vi "PH_Sequencer_Watch.PC _SetVoltage.vi"(0 "i ref in":refnum<vi>, 2 "Tagname":string, 3 "Tagvalue":dbl, 5 "error in (no error)":errorcluster) -> (14 "i ref out":refnum<vi>, 19 "error out":errorcluster)   [LabVIEW 2014, in "PH_Sequencer_Watch.lvlib"]
doc: "This VI writes the incoming information for the voltage to be applied to the related GUI element."
uses:
  PH_Sequencer_Watch.lvlib
  PH_PP_Common/PH_PP_Common.PSU Tags.ctl
  PH_PP_Common/PH_PP_Common.lvlib
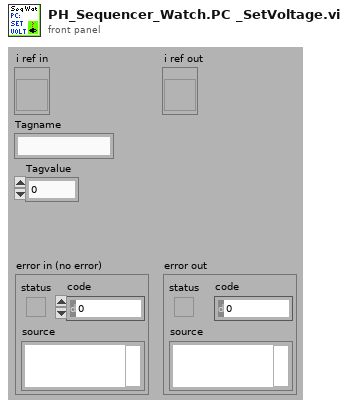
[diagram p1: front panel]
types:
  T1 = typedef "PH_Sequencer_Watch.lvlib/PH_Sequencer_Watch.i attribute.ctl" = cluster{"GUI Refs":cluster{"Shot ID":refnum<vi>, "Sequencer SM State":refnum<vi>, "Remaining Time":refnum<vi>, "PHELIX_Timing_T2":refnum<vi>, "T2-Unit-Dummy":refnum<vi>, "fs_Synchrolock_Watch":refnum<vi>, "Experiment_Vacuum_Control_Experiment":refnum<vi>}, "Status Synchrolock":T2, "Exp - Pressure":dbl, "Exp - Limit":dbl, "Heads":T3[], "Refs BooleanState":refnum<vi>[]}
  T2 = typedef "PH_StatusHandler.lvlib/PH_StatusHandler.Status.ctl" = i16
  T3 = typedef "PH_Sequencer_Watch.lvlib/PH_Sequencer_Watch.Head Information.ctl" = cluster{"Ref Volt":refnum<vi>, "PU":T4}
  T4 = typedef "PH_PP_Common.lvlib/PH_PP_Common.PUs.ctl" = enum16{"no Info", "PA-19mm-1", "PA-19mm-2", "PA-45mm-PILC", "PA-45mm-MAIN", "MA-PU-1", "MA-PU-2", "MA-PU-3", "MA-PU-4", "MA-PU-5", "MA-PU-6", "MA-FR", "MA-PILC", "PA-45mm-DP"}
  T5 = typedef "PH_PP_Common.lvlib/PH_PP_Common.PSU Tags.ctl" = enum16{"voltage-indicator", "peak-detect", "current", "voltage", "inihibit-indicator", "end-of-charge", "HV-on-indicator", "overtemperature", "interlock-indicator", "load-fault", "sum-fault", "HV-off-indicator", "DC-ok", "inhibit", "HV-on", "interlock", "reset", "Status", "Limits"}
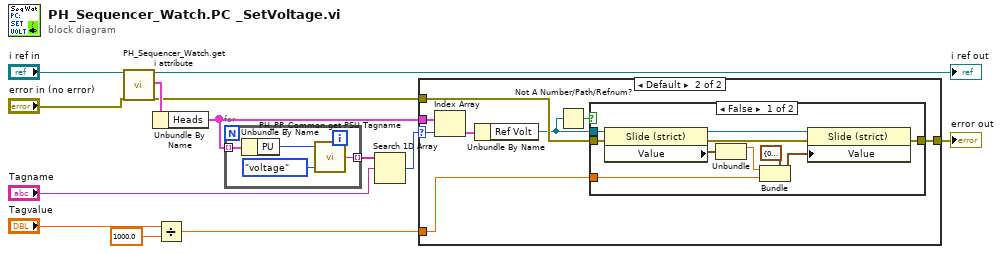
[diagram p0: block diagram]
diagram:
  n1 = call "PH_Sequencer_Watch.get i attribute.vi"("i ref in"="i ref in", "error in (no error)"="error in (no error)") -> ("i ref out"=→"i ref out":refnum<vi>, "i attribute"=w12:T1, "error out"=w11:errorcluster)  [unwired: 15 in]
  n2 = Unbundle By Name(w12) -> ("Heads"=w10:T3[])
  n3 = Divide(x="Tagvalue", y=1000.0) -> (x/y=w5:dbl)
  n4 = for {
    tunnel: w10 -> [w17] mode=indexing
    tunnel: [w15] -> w9 mode=indexing
    n5 = Unbundle By Name(w17) -> ("PU"=w16:T4)
    n6 = call "PH_PP_Common.get PSU Tagname.vi"("PSU Tag"=PH_PP_Common.PSU_Tags."voltage", "PU"=w16) -> ("PSU Tagname"=w15:string)  [unwired: 1 in]
  }
  n7 = Search 1D Array(1D array=w9, element="Tagname") -> (index of element=w8:i32)  [unwired: 1 in]
  n8 = case shown="Default" w8 {
    selector: w8 -> [_ w19]
    tunnel: [w18 w26] -> w6
    tunnel: w5 -> [_ w25]
    tunnel: w11 -> [w18 w24]
    tunnel: w10 -> [_ w23]
    frame -1 {
    }
    frame Default {
      n9 = Index Array(array=w23, index=w19) -> (element=w21:T3)
      n10 = Unbundle By Name(w21) -> ("Ref Volt"=w20:refnum<vi>)
      n11 = Not A Number/Path/Refnum?(number/path/refnum=w20) -> (NaN/Path/Refnum?=w22:bool)
      n12 = case shown="False" w22 {
        tunnel: w20 -> [w32 _]
        tunnel: w24 -> [w35 w37]
        tunnel: [w34 w37] -> w26
        tunnel: w25 -> [w27 _]
        frame False {
          n13 = property class="Slide (strict)"(reference=w32, error in=w35) -> (reference out=w33:refnum<vi>, error out=w36:errorcluster, "Value"=w31:cluster{dbl, dbl})
          n14 = Unbundle(w31) -> (w28:dbl)  [unwired: 1 out]
          n15 = Bundle(cluster=cluster{dbl, dbl} {0.0, 0.0} ("Value"), w28, w27) -> (w30:cluster{dbl, dbl})
          n16 = property class="Slide (strict)"(reference=w33, error in=w36, "Value"=w30) -> (error out=w34:errorcluster)  [unwired: 1 out]
        }
        frame True {
        }
      }
    }
  }
  "error out" <- w6
